vi "adaptPosEstBall.vi"(4 "AttakingOurselves":bool, 6 "Utilities.lvclass":refnum<class "Utilities.lvclass">, 8 "error in (no error)":errorcluster, 9 "Robot":refnum<class "Robot.lvclass">, 10 "BallRef":refnum<class "Ball.lvclass">, 11 "KickToSkill in":refnum<class "KickToSkill.lvclass">) -> (0 "error out":errorcluster, 2 "Pos_est adapted":dbl[](array[numeric]), 3 "KickToSkill out":refnum<class "KickToSkill.lvclass">)   [LabVIEW 2023, in "KickToSkill.lvclass"]
uses:
  KickToSkill.lvclass
  Ball_class/Ball.lvclass
  C:/Users/roboi/Downloads/VSS_AI-Larc2023 - Copia (2)/Object_class/Object.lvclass
  Robot_class/Robot.lvclass
  Utilities_class/Utilities.lvclass
  Object_class/Object.lvclass/Object.ctl
  Object_class/Read x.vi
  Object_class/Read y.vi
  Object_class/Read pos_est_x.vi
  Object_class/Read pos_est_y.vi
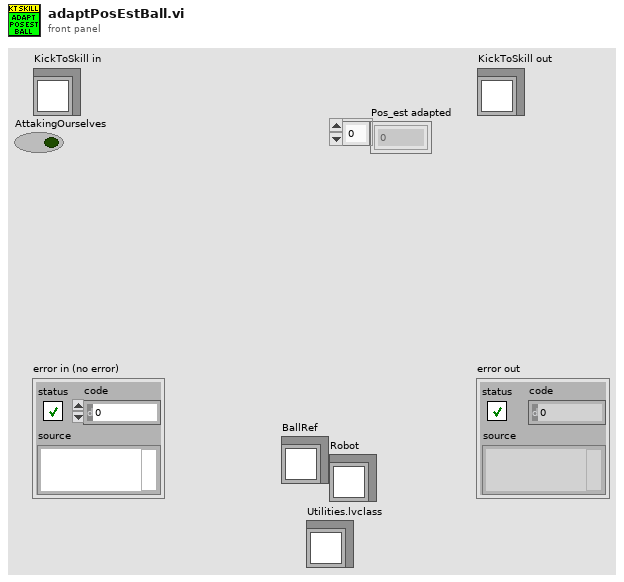
[diagram p1: front panel]
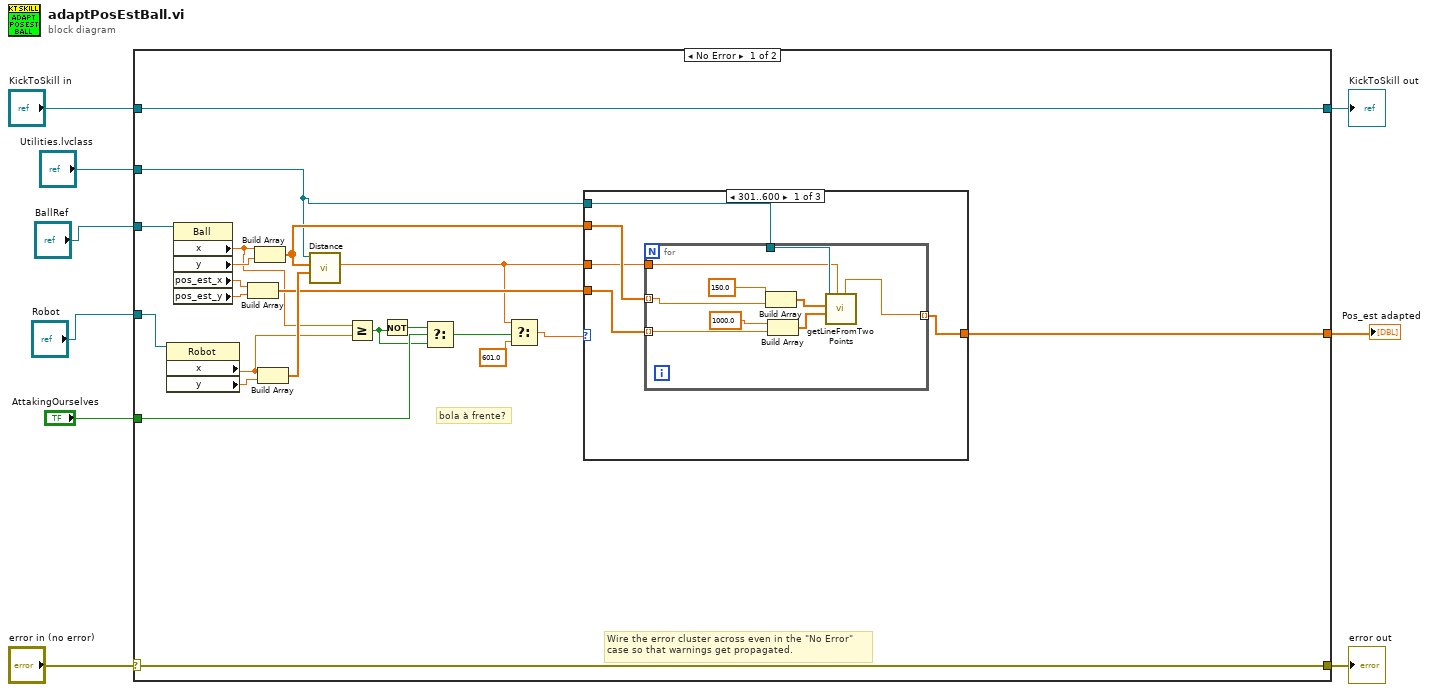
[diagram p0: block diagram]
diagram:
  n1 = case shown="No Error" "error in (no error)" {
    selector: "error in (no error)" -> [w30 w49]
    tunnel: [w30 w49] -> w8
    tunnel: [w31 w48] -> w6
    tunnel: "KickToSkill in" -> [w31 w48]
    tunnel: "BallRef" -> [w29 _]
    tunnel: "Robot" -> [w28 _]
    tunnel: "Utilities.lvclass" -> [w19 _]
    tunnel: [w24 _] -> w2
    tunnel: "AttakingOurselves" -> [w13 _]
    frame No Error {
      # "bola à frente?"
      # "Wire the error cluster across even in the \"No Error\"\ncase so that warnings get propagated."
      n2 = property class="Robot"(reference=w28) -> ("x"=w17:dbl, "y"=w26:dbl)  [unwired: 1 in, 2 out]
      n3 = property class="Ball"(reference=w29) -> ("x"=w18:dbl, "y"=w27:dbl, "pos_est_x"=w22:dbl, "pos_est_y"=w21:dbl)  [unwired: 1 in, 2 out]
      n4 = Build Array(w22, w21) -> (w20:dbl[])
      n5 = Build Array(w18, w27) -> (w23:dbl[])
      n6 = Build Array(w17, w26) -> (w25:dbl[])
      n7 = call "Distance.vi"("P1"=w25, "P2"=w23, "Utilities in"=w19) -> ("Distance"=w16:dbl)  [unwired: 6 in, 2 out]
      n8 = Greater Or Equal?(x=w18, y=w17) -> (x >= y?=w12:bool)
      n9 = Not(x=w12) -> (.not. x?=w11:bool)
      n10 = Select(t=w11, s=w13, f=w12) -> (s? t:f=w10:bool)
      n11 = Select(t=w16, s=w10, f=601.0) -> (s? t:f=w15:dbl)
      n12 = case shown="301..600" w15 {
        tunnel: [w32 w46 w47] -> w24
        tunnel: w23 -> [w35 _ w47]
        tunnel: w20 -> [w34 w46 _]
        tunnel: w19 -> [w36 _ _]
        tunnel: w16 -> [w33 _ _]
        frame 301..600 {
          n13 = for {
            tunnel: w36 -> [w45]
            tunnel: w35 -> [w42] mode=indexing
            tunnel: w34 -> [w41] mode=indexing
            tunnel: w33 -> [w38]
            tunnel: [w37] -> w32 mode=indexing
            n14 = Build Array(150.0, w42) -> (w40:dbl[])
            n15 = Build Array(1000.0, w41) -> (w39:dbl[])
            n16 = call "getLineFromTwoPoints.vi"("x informed (optional)"=w38, "Point 2"=w39, "Point 1"=w40, "Utilities in"=w45) -> ("y to x informed (opitional)"=w37:dbl)  [unwired: 3 in, 4 out]
          }
        }
        frame Default {
          # "Dist maior que 600"
        }
        frame 0..300 {
        }
      }
    }
    frame Error {
    }
  }
  "error out" <- w8
  "KickToSkill out" <- w6
  "Pos_est adapted" <- w2
